vi "Write.vi"(8 "error in (no error)":errorcluster, 9 "Variant":variant, 10 "String":string, 11 "GPIB in":refnum<class "GPIB.lvclass">) -> (0 "error out":errorcluster, 3 "GPIB out":refnum<class "GPIB.lvclass">)   [LabVIEW 2013, in "GPIB.lvclass"]
uses:
  GPIB.lvclass
  VISA/VISA.lvclass/VISA.ctl
  VISA/Read Ref.vi
  VISA/Write Ref.vi
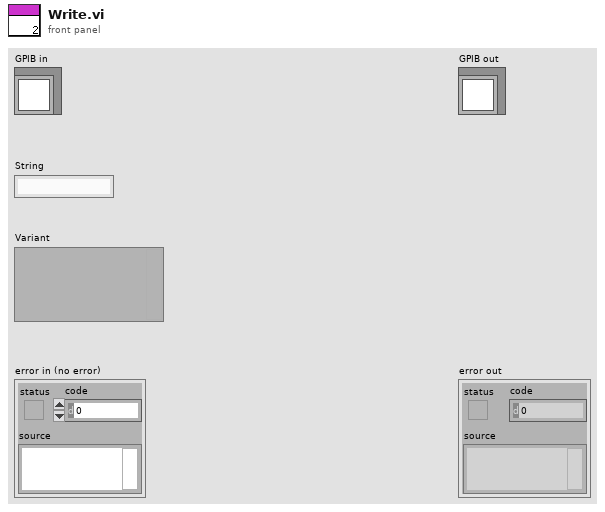
[diagram p1: front panel]
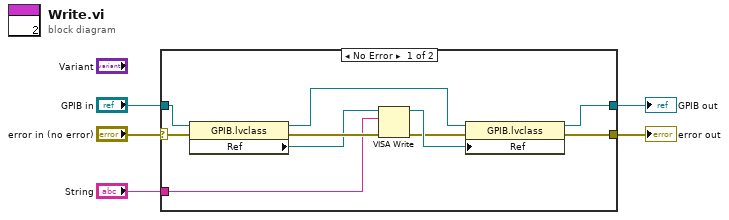
[diagram p0: block diagram]
diagram:
  n1 = case shown="No Error" "error in (no error)" {
    selector: "error in (no error)" -> [w6 w17]
    tunnel: "GPIB in" -> [w15 w16]
    tunnel: "String" -> [w13 _]
    tunnel: [w9 w17] -> w2
    tunnel: [w7 w16] -> w1
    frame No Error {
      n2 = property class="GPIB.lvclass"(reference=w15, error in=w6) -> (reference out=w8:refnum<class "GPIB.lvclass">, error out=w14:errorcluster, "Ref"=w12:refnum<visa-resource-name>)
      n3 = VISA Write(VISA resource name=w12, write buffer=w13, error in (no error)=w14) -> (VISA resource name out=w11:refnum<visa-resource-name>, error out=w10:errorcluster)  [unwired: 1 out]
      n4 = property class="GPIB.lvclass"(reference=w8, error in=w10, "Ref"=w11) -> (reference out=w7:refnum<class "GPIB.lvclass">, error out=w9:errorcluster)
    }
    frame Error {
    }
  }
  "error out" <- w2
  "GPIB out" <- w1
